vi "Add Industrial Controller.vi"(8 "error in (no error)":errorcluster, 11 "Node Ptr":u64 format="%.0x") -> (0 "error out":errorcluster, 2 "Parameters Ref out":T1 format="%.0x", 3 "Controller Ref out":T1 format="%.0x")   [LabVIEW 2019, in "Control Addon Shared.lvlib"]
uses:
  Control Addon Shared.lvlib
  <vilib>/NI VeriStand/Custom Device API/Custom Device Item Ref.ctl
  <vilib>/NI VeriStand/Custom Device API/Custom Device Channel.ctl
  <vilib>/NI VeriStand/Custom Device API/Custom Device Channel Type.ctl
  Types/Action.ctl
  Types/Controller Settings.ctl
  Constants.vi
  <vilib>/NI VeriStand/Custom Device API/NI VeriStand - Get Item Property.vi
  <vilib>/NI VeriStand/Custom Device API/Get Item Property (Double).vi
  <vilib>/NI VeriStand/Custom Device API/Get Item Property (Boolean).vi
  <vilib>/NI VeriStand/Custom Device API/NI VeriStand - Set Item Property.vi
  <vilib>/NI VeriStand/Custom Device API/Set Item Property (Double).vi
  <vilib>/NI VeriStand/Custom Device API/Set Item Property (Boolean).vi
  <vilib>/NI VeriStand/Custom Device API/Custom Device API.lvlib
panel:
  in  "Tag":string
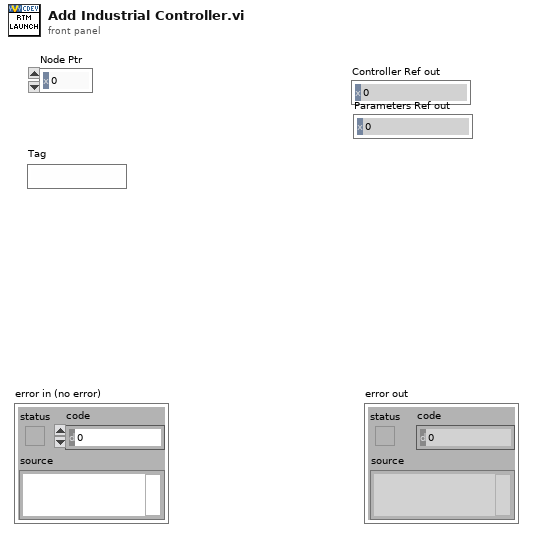
[diagram p1: front panel]
types:
  T1 = typedef "Custom Device API.lvlib/Custom Device Item Ref.ctl" = u64
  T2 = typedef "Control Addon Shared.lvlib/Controller Settings.ctl" = cluster{"Output Max":dbl, "Output Min":dbl, "Setpoint Max":dbl, "Setpoint Min":dbl, "Use External Setpoint":bool, "Output Rate Limiter":dbl}
  T3 = typedef "Control Addon Shared.lvlib/Action.ctl" = enum16{"Get", "Set"}
  T4 = typedef "Custom Device API.lvlib/Custom Device Channel.ctl" = cluster{"Type":T5, "Units":string, "Default Value":dbl, "Faultable":bool, "Scalable":bool}
  T5 = typedef "Custom Device API.lvlib/Custom Device Channel Type.ctl" = enum16{"Input", "Output"}
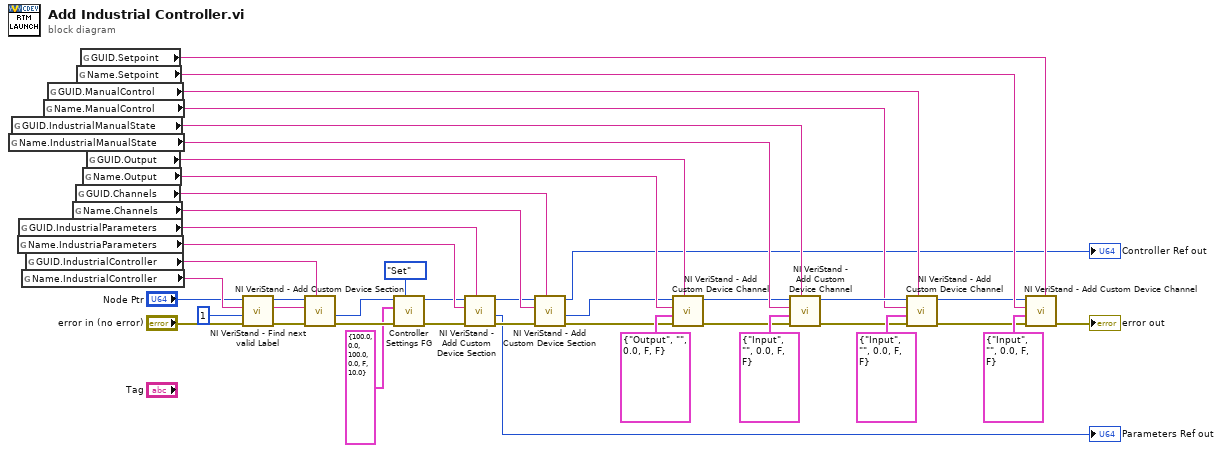
[diagram p0: block diagram]
diagram:
  n1 = global read "Constants.vi" "Name.IndustrialManualState"() -> (w19:string)
  n2 = global read "Constants.vi" "GUID.IndustrialManualState"() -> (w15:string)
  n3 = global read "Constants.vi" "Name.IndustriaParameters"() -> (w40:string)
  n4 = global read "Constants.vi" "GUID.IndustrialParameters"() -> (w39:string)
  n5 = global read "Constants.vi" "Name.IndustrialController"() -> (w36:string)
  n6 = global read "Constants.vi" "GUID.IndustrialController"() -> (w43:string)
  n7 = global read "Constants.vi" "Name.ManualControl"() -> (w18:string)
  n8 = global read "Constants.vi" "GUID.ManualControl"() -> (w17:string)
  n9 = global read "Constants.vi" "Name.Channels"() -> (w27:string)
  n10 = global read "Constants.vi" "GUID.Channels"() -> (w28:string)
  n11 = global read "Constants.vi" "Name.Setpoint"() -> (w37:string)
  n12 = global read "Constants.vi" "GUID.Setpoint"() -> (w14:string)
  n13 = global read "Constants.vi" "Name.Output"() -> (w38:string)
  n14 = global read "Constants.vi" "GUID.Output"() -> (w16:string)
  n15 = call <vilib>:"NI VeriStand - Find next valid Label.vi"("error in (no error)"="error in (no error)", "Start Value (1)"=1, "Label"=w36, "Item Ref in"="Node Ptr") -> ("error out"=w31:errorcluster, "Label out"=w35:string, "Item Ref out"=w33:T1)  [unwired: 3 in, 2 out]
  n16 = call <vilib>:"NI VeriStand - Add Custom Device Section.vi"("GUID (Default Section)"=w43, "error in (no error)"=w31, "Section Name"=w35, "Parent Ref in"=w33) -> ("error out"=w5:errorcluster, "Section Ptr"=w4:T1)  [unwired: 4 in, 2 out]
  n17 = call "Controller Settings FG.vi"("Action"=Action."Set", "error in (no error)"=w5, "Controller Settings"=T2 {"Output Max"=100.0, "Output Min"=0.0, "Setpoint Max"=100.0, "Setpoint Min"=0.0, "Use External Setpoint"=FALSE, "Output Rate Limiter"=10.0}, "Node Ptr"=w4) -> ("error out"=w2:errorcluster, "Item Ref out"=w3:T1)  [unwired: 5 in, 1 out]
  n18 = call <vilib>:"NI VeriStand - Add Custom Device Section.vi"("GUID (Default Section)"=w39, "error in (no error)"=w2, "Section Name"=w40, "Parent Ref in"=w3) -> ("error out"=w24:errorcluster, "Section Ptr"=→"Parameters Ref out":T1, "Parent Ref out"=w25:T1)  [unwired: 4 in, 1 out]
  n19 = call <vilib>:"NI VeriStand - Add Custom Device Section.vi"("GUID (Default Section)"=w28, "error in (no error)"=w24, "Section Name"=w27, "Parent Ref in"=w25) -> ("error out"=w30:errorcluster, "Section Ptr"=w29:T1, "Parent Ref out"=→"Controller Ref out":T1)  [unwired: 4 in, 1 out]
  n20 = call <vilib>:"NI VeriStand - Add Custom Device Channel.vi"("GUID (Default Channel)"=w16, "error in (no error)"=w30, "Channel"=T4 {"Type"=enum."Output", "Units"="", "Default Value"=0.0, "Faultable"=FALSE, "Scalable"=FALSE}, "Channel Name"=w38, "Parent Ref in"=w29) -> ("error out"=w12:errorcluster, "Parent Ref out"=w13:T1)  [unwired: 3 in, 2 out]
  n21 = call <vilib>:"NI VeriStand - Add Custom Device Channel.vi"("GUID (Default Channel)"=w15, "error in (no error)"=w12, "Channel"=T4 {"Type"=enum."Input", "Units"="", "Default Value"=0.0, "Faultable"=FALSE, "Scalable"=FALSE}, "Channel Name"=w19, "Parent Ref in"=w13) -> ("error out"=w21:errorcluster, "Parent Ref out"=w20:T1)  [unwired: 3 in, 2 out]
  n22 = call <vilib>:"NI VeriStand - Add Custom Device Channel.vi"("GUID (Default Channel)"=w17, "error in (no error)"=w21, "Channel"=T4 {"Type"=enum."Input", "Units"="", "Default Value"=0.0, "Faultable"=FALSE, "Scalable"=FALSE}, "Channel Name"=w18, "Parent Ref in"=w20) -> ("error out"=w10:errorcluster, "Parent Ref out"=w9:T1)  [unwired: 3 in, 2 out]
  n23 = call <vilib>:"NI VeriStand - Add Custom Device Channel.vi"("GUID (Default Channel)"=w14, "error in (no error)"=w10, "Channel"=T4 {"Type"=enum."Input", "Units"="", "Default Value"=0.0, "Faultable"=FALSE, "Scalable"=FALSE}, "Channel Name"=w37, "Parent Ref in"=w9) -> ("error out"=→"error out":errorcluster)  [unwired: 3 in, 3 out]
